vi "get_root_table.vi"(8 "error in (no error)":errorcluster, 11 "Doc in":refnum<class "Doc.lvclass">) -> (0 "error out":errorcluster, 1 "Table":refnum<class "Table.lvclass">, 3 "Doc out":refnum<class "Doc.lvclass">)   [LabVIEW 2020, in "toml_edit.lvlib" / "Doc.lvclass"]
uses:
  Doc.lvclass
  Doc.lvclass/Doc.ctl
  Table/Table.lvclass
  dragon_toml_64.dll
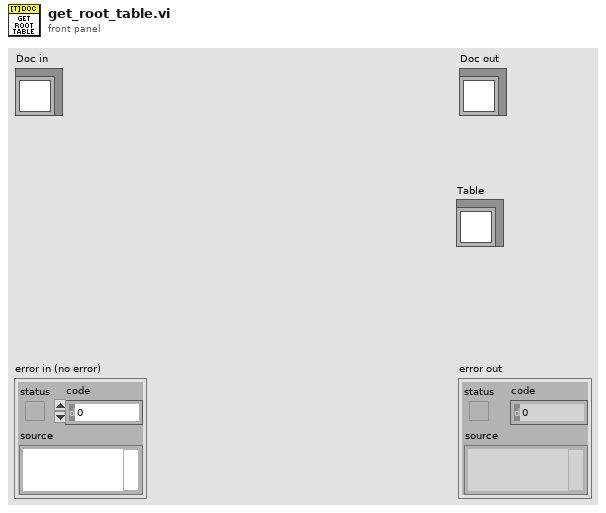
[diagram p1: front panel]
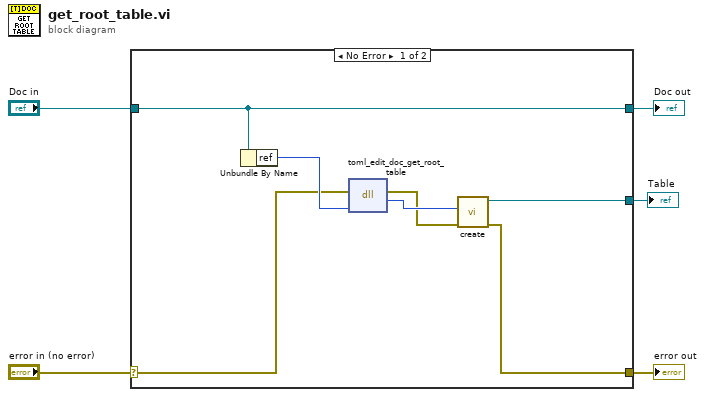
[diagram p0: block diagram]
diagram:
  n1 = case shown="No Error" "error in (no error)" {
    selector: "error in (no error)" -> [w10 w14]
    tunnel: [w6 w14] -> w4
    tunnel: [w11 w13] -> w2
    tunnel: "Doc in" -> [w11 w13]
    tunnel: [w7 _] -> w1
    frame No Error {
      n2 = Unbundle By Name(w11) -> ("ref"=w12:u64)
      n3 = dll-call lib="C:/Projects/toml-edit-labview/lv_src/dragon_toml_*.dll" fn="toml_edit_doc_get_root_table"(error in=w10, "doc_ref"=w12) -> (error out=w8:errorcluster, "table_ptr"=w9:u64)  [unwired: 3 in, 1 out]
      n4 = call "create.vi"("error in (no error)"=w8, "ref"=w9) -> ("error out"=w6:errorcluster, "Table out"=w7:refnum<class "Table.lvclass">)  [unwired: 8 in]
    }
    frame Error {
    }
  }
  "error out" <- w4
  "Doc out" <- w2
  "Table" <- w1
